vi "LCP Is Enabled.vi"(8 "error in (no error)":errorcluster caption="Fehler (Eingang, kein Fehler)", 11 "Pump Handle":i64) -> (0 "error out":errorcluster caption="Fehler (Ausgang)", 3 "Enabled":bool)   [LabVIEW 2021, in "labbCAN_Pump_API.lvlib"]
doc: "LCP_Func long LCP_CALL LCP_IsEnabled(dev_hdl hPump);"
uses:
  labbCAN_Pump_API.lvlib
  labbCAN_Pump_API.dll
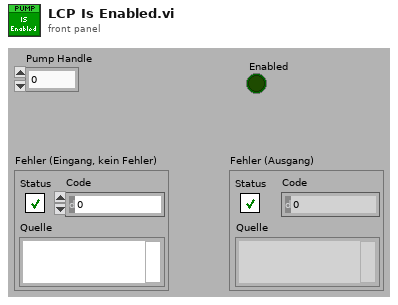
[diagram p1: front panel]
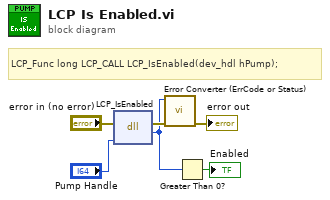
[diagram p0: block diagram]
diagram:
  # "LCP_Func long LCP_CALL LCP_IsEnabled(dev_hdl hPump);"
  n1 = dll-call lib="C:/Users/olaja/AppData/Local/CETONI_SDK/labbCAN_Pump_API.*" fn="LCP_IsEnabled"(error in="error in (no error)", "hPump"="Pump Handle") -> (error out=w4:errorcluster, "Rückgabetyp"=w1:i32)  [unwired: 3 in, 1 out]
  n2 = call "Error Converter (ErrCode or Status).vi"("error in (no error)"=w4, "error code"=w1) -> ("error out"=→"error out":errorcluster)  [unwired: 9 in]
  n3 = Greater Than 0?(x=w1) -> (x > 0?=→"Enabled":bool)
